vi "Do.vi"(8 "error in (no error)":errorcluster, 10 "Actor in":refnum<class "Actor.lvclass">, 11 "Rcv Caller Notice Msg":refnum<class "Rcv Caller Notice Msg.lvclass">) -> (0 "error out":errorcluster, 2 "Actor out":refnum<class "Actor.lvclass">)   [LabVIEW 2020, in "Generic Actor.lvlib" / "Rcv Caller Notice Msg.lvclass"]
doc: "This VI delivers the message to the actor by calling the appropriate method(s) on the actor."
uses:
  Rcv Caller Notice Msg.lvclass
  E:/NI I Program/Actor FCT Frame/Generic Actor/Generic Actor Messages/Caller Notice Msg/Caller Notice Msg.lvclass
  <vilib>/ActorFramework/Actor/Actor.lvclass
  Generic Actor/Generic Actor.lvclass
  C:/Program Files (x86)/National Instruments/LabVIEW 2020/vi.lib/ActorFramework/Actor/Actor.lvclass
  Caller Notice Msg/Caller Notice Msg.lvclass/Caller Notice Msg.ctl
  b313a96b-00c4-4189-8544-d4de435bfb11.vi
  Caller Notice Msg/Caller Notice Msg.lvclass
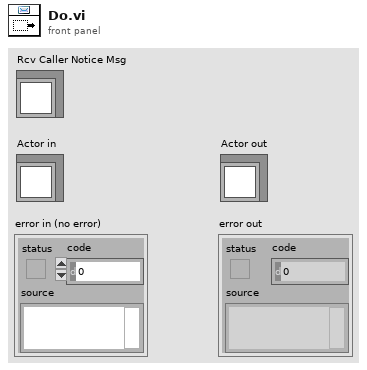
[diagram p1: front panel]
types:
  T1 = cluster{"Actor Name":string, "Action Name":string, "Params":variant}
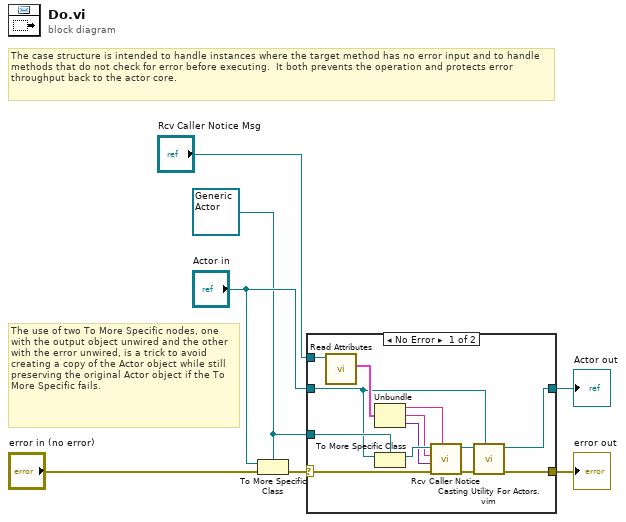
[diagram p0: block diagram]
diagram:
  w2 = refnum<class "Generic Actor.lvclass"> refnum ("Actor in")
  # "The use of two To More Specific nodes, one with the output object unwired and the other with the error unwired, is a trick to avoid creating a copy of the Actor object while still preserving the original Actor object if the To More Specific fails."
  # "The case structure is intended to handle instances where the target method has no error input and to handle methods that do not check for error before executing.  It both prevents the operation and protects error throughput back to the actor core."
  n1 = To More Specific Class(target class=w2, reference="Actor in", error in="error in (no error)") -> (error out=w1:errorcluster)  [unwired: 1 out]
  n2 = case shown="No Error" w1 {
    selector: w1 -> [w20 w22]
    tunnel: [w13 w22] -> w7
    tunnel: [w12 w21] -> w6
    tunnel: "Actor in" -> [w16 w21]
    tunnel: w2 -> [w17 _]
    tunnel: "Rcv Caller Notice Msg" -> [w18 _]
    frame No Error {
      n3 = call "Read Attributes.vi"("Caller Notice Msg"=w18) -> ("Payload"=w19:T1)  [unwired: 10 in]
      n4 = Unbundle(w19) -> ("Actor Name"=w10:string, "Action Name"=w9:string, "Params"=w8:variant)
      n5 = To More Specific Class(target class=w17, reference=w16) -> (specific class reference=w11:refnum<class "Generic Actor.lvclass">)  [unwired: 1 in, 1 out]
      n6 = call-dynamic "Rcv Caller Notice.vi"("Actor Name"=w10, "error in (no error)"=w20, "Params"=w8, "Action Name"=w9, "Generic Actor in"=w11) -> ("error out"=w14:errorcluster, "Generic Actor out"=w15:refnum<class "Generic Actor.lvclass">)  [unwired: 5 in]
      n7 = call "Casting Utility For Actors.vim"("type"=w16, "error in (no error)"=w14, "Actor in"=w15) -> ("error out"=w13:errorcluster, "Actor out"=w12:refnum<class "Actor.lvclass">)  [unwired: 7 in]
    }
    frame Error {
      # "If type check fails, pass the original object out again."
    }
  }
  "error out" <- w7
  "Actor out" <- w6
